vi "Text lines to string array.vi"(8 "error in (no error)":errorcluster, 11 "String":string) -> (0 "error out":errorcluster, 3 "String array":string[](array[string]))   [LabVIEW 2013]
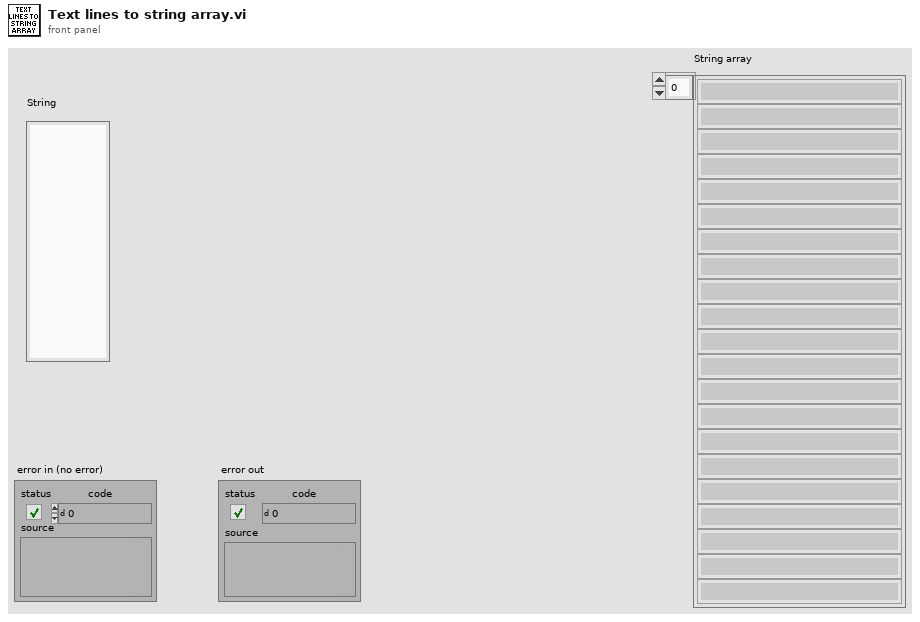
[diagram p1: front panel]
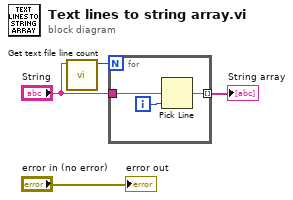
[diagram p0: block diagram]
diagram:
  n1 = call "Get text file line count.vi"("text string"="String") -> ("Line cnt"=w3:i32)  [unwired: 9 in, 1 out]
  n2 = for {
    N: w3 -> [_]
    tunnel: "String" -> [w6]
    tunnel: [w5] -> w1 mode=indexing
    i -> [w7]
    n3 = Pick Line(multi-line string=w6, line index=w7) -> (output string=w5:string)  [unwired: 1 in]
  }
  "String array" <- w1
  "error out" <- "error in (no error)"
